vi "get voltage range byte.vi"(8 "error in (no error)":errorcluster caption="에러 입력(에러 없음)", 10 "voltage range":dbl, 11 "DW7802 입력":refnum<class "DW7802.lvclass">) -> (0 "error out":errorcluster caption="에러 출력", 2 "byte value":u8 format="%02x", 3 "DW7802 출력":refnum<class "DW7802.lvclass">)   [LabVIEW 2020, in "DW7802.lvclass"]
uses:
  DW7802.lvclass
  73e844e5-ec43-47e8-a19a-c44a7a3cf020.vi
  <vilib>/Comparison/Equal/Equal Functor/Equal Functor.lvclass
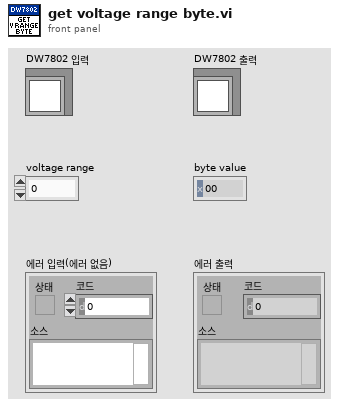
[diagram p1: front panel]
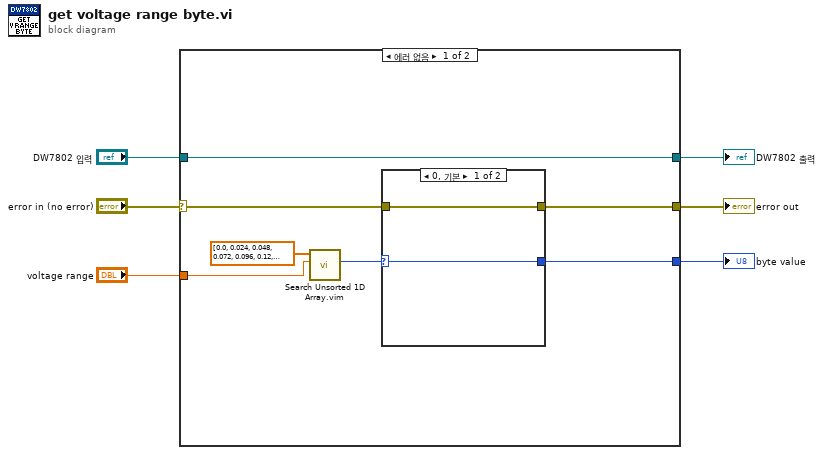
[diagram p0: block diagram]
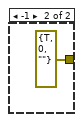
[diagram p2: hidden frame]
diagram:
  n1 = case shown="에러 없음" "error in (no error)" {
    selector: "error in (no error)" -> [w10 w18]
    tunnel: [w7 w18] -> w6
    tunnel: "DW7802 입력" -> [w13 w17]
    tunnel: [w13 w17] -> w4
    tunnel: "voltage range" -> [w11 _]
    tunnel: [w8 _] -> w5
    frame No Error {
      n2 = call "Search Unsorted 1D Array.vim"("element"=w11, "unsorted 1D array"=dbl[] [0.0, 0.024, 0.048, 0.072, 0.096, 0.12, 0.144, 0.168, 0.192, 0.216, 0.24, 0.264, 0.288, 0.312, 0.336, 0.36, 0.384, 0.408, 0.432, 0.456, 0.48, 0.504, 0.528, 0.552, 0.576, 0.6, 0.624, 0.648, 0.672, 0.696, 0.72, 0.744, 0.768, 0.792, 0.816, 0.84, 0.864, 0.888, 0.912, 0.936, 0.96, 0.984, 1.008, 1.032, 1.056, 1.08, 1.104, 1.128, 1.152, 1.176, 1.2, 1.224, 1.248, 1.272, 1.296, 1.32, 1.344, 1.368, 1.392, 1.416, 1.44, 1.464, 1.488, 1.512, 1.536, 1.56, 1.584, 1.608, 1.632, 1.656, 1.68, 1.704, 1.728, 1.752, 1.776, 1.8, 1.824, 1.848, 1.872, 1.896, 1.92, 1.944, 1.968, 1.992, 2.016, 2.04, 2.064, 2.088, 2.112, 2.136, 2.16, 2.184, 2.208, 2.232, 2.256, 2.28, 2.304, 2.328, 2.352, 2.376, 2.4, 2.424, 2.448, 2.472, 2.496, 2.52, 2.544, 2.568, 2.592, 2.616, 2.64, 2.664, 2.688, 2.712, 2.736, 2.76, 2.784, 2.808, 2.832, 2.856, 2.88, 2.904, 2.928, 2.952, 2.976, 3.0, 3.024, 3.048, 3.072, 3.096, 3.12, 3.144, 3.168, 3.192, 3.216, 3.24, 3.264, 3.288, 3.312, 3.336, 3.36, 3.384, 3.408, 3.432, 3.456, 3.48, 3.504, 3.528, 3.552, 3.576, 3.6, 3.624, 3.648, 3.672, 3.696, 3.72, 3.744, 3.768, 3.792, 3.816, 3.84, 3.864, 3.888, 3.912, 3.936, 3.96, 3.984, 4.008, 4.032, 4.056, 4.08, 4.104, 4.128, 4.152, 4.176, 4.2, 4.224, 4.248, 4.272, 4.296, 4.32, 4.344, 4.368, 4.392, 4.416, 4.44, 4.464, 4.488, 4.512, 4.536, 4.56, 4.584, 4.608, 4.632, 4.656, 4.68, 4.704, 4.728, 4.752, 4.776, 4.8, 4.824, 4.848, 4.872, 4.896, 4.92, 4.944, 4.968, 4.992, 5.016, 5.04, 5.064, 5.088, 5.112, 5.136, 5.16, 5.184, 5.208, 5.232, 5.256, 5.28, 5.304, 5.328, 5.352, 5.376, 5.4, 5.424, 5.448, 5.472, 5.496, 5.52, 5.544, 5.568, 5.592, 5.616, 5.64, 5.664, 5.688, 5.712, 5.736, 5.76, 5.784, 5.808, 5.832, 5.856, 5.88, 5.904, 5.928, 5.952, 5.976, 6.0, 6.024, 6.048, 6.072, 6.096, 6.12]) -> ("index of element"=w9:i32)  [unwired: 9 in]
      n3 = case shown="0, 기본" w9 {
        selector: w9 -> [w15 _]
        tunnel: w10 -> [w14 _]
        tunnel: [w15 _] -> w8
        tunnel: [w14 errorcluster {"status"=TRUE, "code"=0, "source"=""} ("error IO")] -> w7
        frame 0, Default {
        }
        frame -1 {
        }
      }
    }
    frame Error {
    }
  }
  "error out" <- w6
  "DW7802 출력" <- w4
  "byte value" <- w5
